vi "GetImages.vi"(4 "File type":T1, 5 "Disabled":bool, 6 "Background Color":u32(colorbox), 7 "image directory":path, 8 "error in":errorcluster, 11 "Knob in":refnum<class "Knob.lvclass">) -> (0 "error out":errorcluster, 3 "Knob out":refnum<class "Knob.lvclass">)   [LabVIEW 2014, in "Raspberry Pi Compatible Compiler for LabVIEW.lvlib" / "Knob.lvclass"]
uses:
  Knob.lvclass
  Control/ImageTypes.ctl
  Raspberry Pi Compatible Compiler for LabVIEW.lvlib
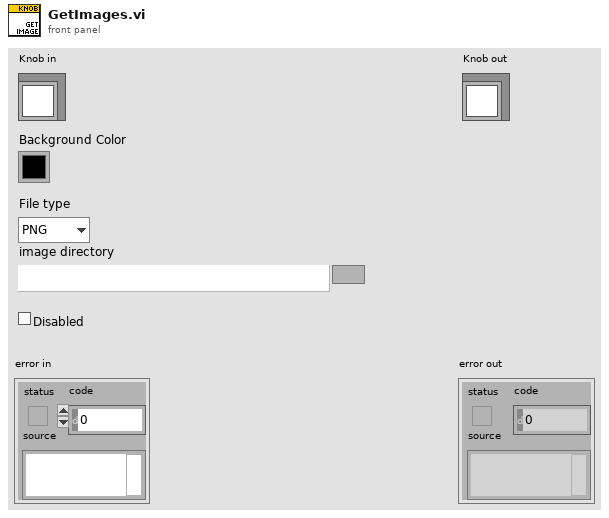
[diagram p1: front panel]
types:
  T1 = typedef "Raspberry Pi Compatible Compiler for LabVIEW.lvlib/ImageTypes.ctl" = enum16{"PNG", "JPEG", "BMP"}
  T2 = typedef "Raspberry Pi Compatible Compiler for LabVIEW.lvlib/KnobTypesTD.ctl" = enum16{"Knob", "Dial", "Meter", "Gauge"}
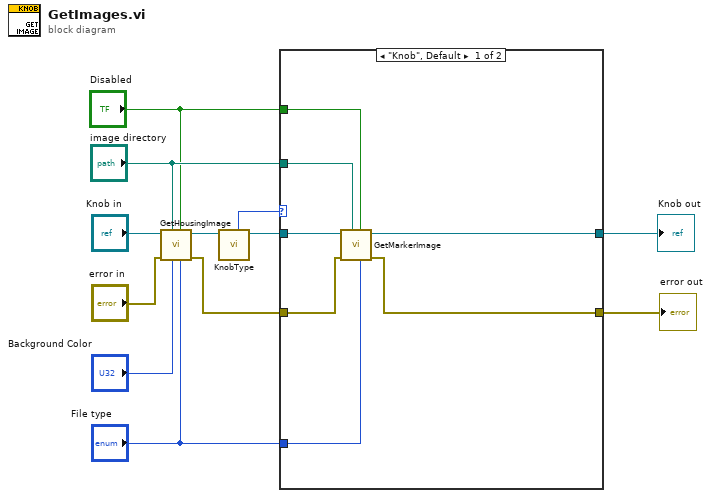
[diagram p0: block diagram]
diagram:
  n1 = call-dynamic "GetHousingImage.vi"("File type"="File type", "Disabled"="Disabled", "Background Color"="Background Color", "image directory"="image directory", "error in"="error in", "Knob in"="Knob in") -> ("error out"=w7:errorcluster, "Knob out"=w11:refnum<class "Knob.lvclass">)  [unwired: 4 in]
  n2 = call "KnobType.vi"("Knob in"=w11) -> ("Knob out"=w8:refnum<class "Knob.lvclass">, "Knob type"=w9:T2)  [unwired: 7 in]
  n3 = case shown="\"Knob\", Default" w9 {
    tunnel: w8 -> [w19 w21]
    tunnel: w7 -> [w16 w20]
    tunnel: "File type" -> [w18 _]
    tunnel: "image directory" -> [w17 _]
    tunnel: [w15 w20] -> w3
    tunnel: [w14 w21] -> w2
    tunnel: "Disabled" -> [w13 _]
    frame "Knob", Default {
      n4 = call-dynamic "GetMarkerImage.vi"("File type"=w18, "Disabled"=w13, "image directory"=w17, "error in"=w16, "Knob in"=w19) -> ("error out"=w15:errorcluster, "Knob out"=w14:refnum<class "Knob.lvclass">)  [unwired: 5 in]
    }
    frame "Dial" {
    }
  }
  "error out" <- w3
  "Knob out" <- w2
